vi "Express SINAD Analyzer.vi"(6 "search (+/- % of fund.)":dbl=5.0 format="%0.2p", 8 "error in (no error)":errorcluster, 9 "approx. fund. freq. (optional)":dbl=-1.0 format="%0.2p", 10 "export signals":T1(ring), 11 "Waveform In":waveform(dbl)[](array[waveform])) -> (0 "error out":errorcluster, 3 "SINAD":waveform(dbl)[](graph), 4 "exported spectrum (dB)":waveform(dbl)[](graph), 5 "exported time signal":waveform(dbl)[](graph))   [LabVIEW 2020]
uses:
  <vilib>/measure/matone.llb/SINAD Analyzer 1 Chan.vi
  <vilib>/measure/NI_MAPro.lvlib
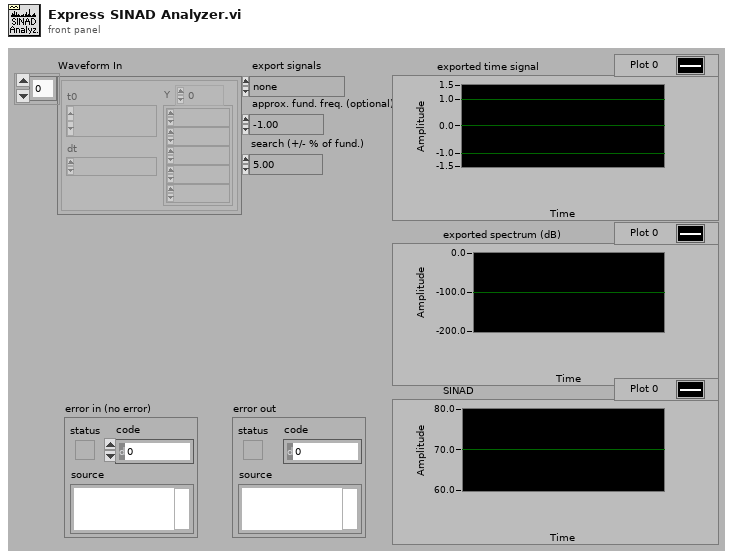
[diagram p1: front panel]
types:
  T1 = enum16{"none", "input signal", "fundamental signal", "residual signal"}
  T2 = cluster{"approx. fund. freq. (optional)":dbl, dbl}
  T3 = cluster{"exported time signal":waveform(dbl), "exported spectrum (dB)":cluster{"f0":dbl, "df":dbl, "dB Spectrum (Hann)":dbl[]}}
  T4 = cluster{"f0":dbl, "df":dbl, "dB Spectrum (Hann)":dbl[]}
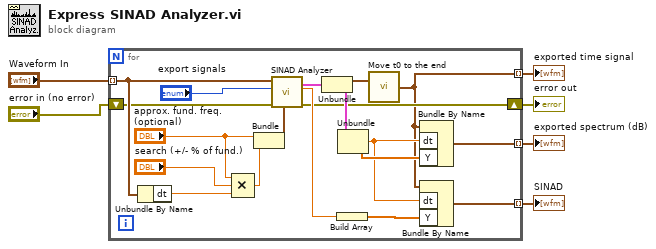
[diagram p0: block diagram]
diagram:
  n1 = for {
    tunnel: "Waveform In" -> [w16] mode=indexing
    tunnel: [w9] -> w6 mode=indexing
    tunnel: [w8] -> w5 mode=indexing
    tunnel: [w7] -> w4 mode=indexing
    shift-right: [w11] -> w1
    shift-left: "error in (no error)" -> [w12]
    n2 = Unbundle By Name(w16) -> ("dt"=w17:dbl)
    n3 = Compound Arithmetic op=MULTIPLY("approx. fund. freq. (optional)", "search (+/- % of fund.)", w17) -> (w13:dbl)
    n4 = Bundle("approx. fund. freq. (optional)"="approx. fund. freq. (optional)", w13) -> (w24:T2)  [unwired: 1 in]
    n5 = call-poly <vilib>:"SINAD Analyzer.vi"("advanced search"=w24, "error in (no error)"=w12, "export  mode"="export signals", "signal in"=w16) -> ("error out"=w11:errorcluster, "SINAD (dB)"=w19:dbl, "exported signals"=w23:T3)  [unwired: 2 in, 3 out]
    n6 = Unbundle(w23) -> ("exported time signal"=w10:waveform(dbl), "exported spectrum (dB)"=w22:T4)
    n7 = Build Array(w19) -> (w20:dbl[])
    n8 = Unbundle(w22) -> ("df"=w18:dbl, "dB Spectrum (Hann)"=w21:dbl[])  [unwired: 1 out]
    n9 = call <vilib>:"Move t0 to the end.vi"("waveform in"=w10) -> ("waveform out"=w9:waveform(dbl))
    n10 = Bundle By Name(cluster=w9, "dt"=w18, "Y"=w21) -> (w8:waveform(dbl))
    n11 = Bundle By Name(cluster=w9, "dt"=w18, "Y"=w20) -> (w7:waveform(dbl))
  }
  "exported time signal" <- w6
  "exported spectrum (dB)" <- w5
  "SINAD" <- w4
  "error out" <- w1
